vi "Utility_Translate circle into Masking ROI.vi"(11 "Fitted Circle":T2) -> (3 "ROI Descriptor":T1)   [LabVIEW 2014]
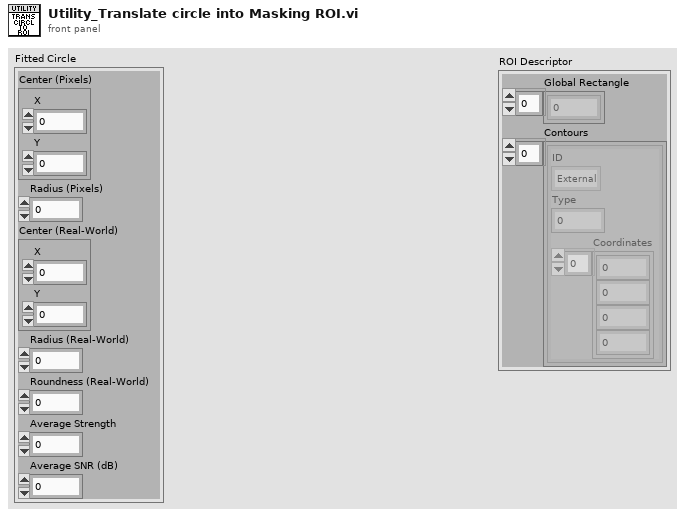
[diagram p1: front panel]
types:
  T1 = cluster{"Global Rectangle":i32[], "Contours":cluster{"ID":enum32{"External", "Internal"}, "Type":u32, "Coordinates":i32[]}[]}
  T2 = cluster{"Center (Pixels)":cluster{"X":sgl, "Y":sgl}, "Radius (Pixels)":dbl, "Center (Real-World)":cluster{"X":sgl, "Y":sgl}, "Radius (Real-World)":dbl, "Roundness (Real-World)":dbl, "Average Strength":dbl, "Average SNR (dB)":dbl}
  T3 = cluster{"ID":enum32{"External", "Internal"}, "Type":u32, "Coordinates":i32[]}
  T4 = cluster{"ID":enum32{"External", "Internal"}, "Type":u32, "Coordinates":i32[]}[]
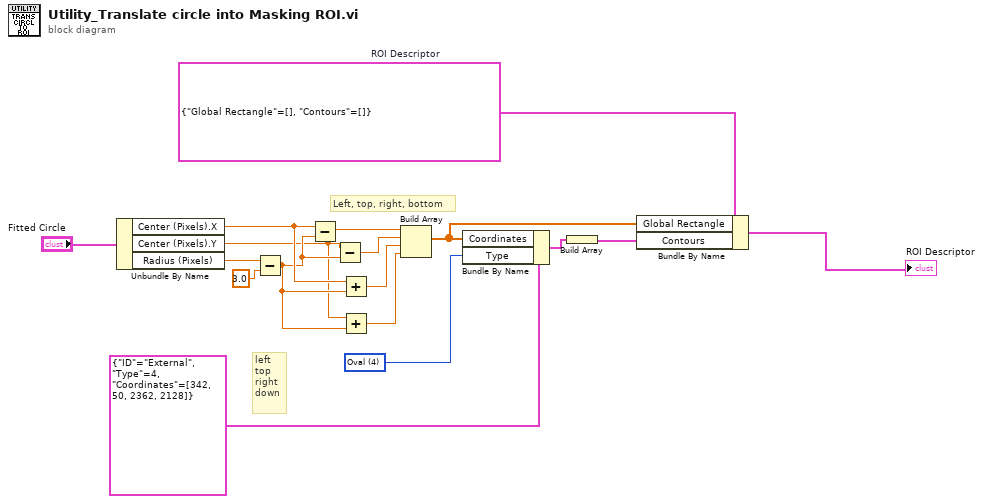
[diagram p0: block diagram]
diagram:
  w1 = u32 4 items=["No Selection", "Point", "Line", "Rectangle", "Oval", "Polygon", "Freehand Region", "Annulus", "Unused2", "Unused3", "Broken Line", "Freehand Line", "Rotated Rectangle"] ("Type")
  w14 = T1 {"Global Rectangle"=[], "Contours"=[]}  # ROI Descriptor
  # "Left, top, right, bottom"
  # "left \ntop\nright \ndown"
  n1 = Unbundle By Name("Fitted Circle") -> ("Center (Pixels).X"=w9:sgl, "Center (Pixels).Y"=w4:sgl, "Radius (Pixels)"=w11:dbl)
  n2 = Subtract(x=w11, y=3.0) -> (x-y=w8:dbl)
  n3 = Subtract(x=w9, y=w8) -> (x-y=w7:dbl)
  n4 = Subtract(x=w4, y=w8) -> (x-y=w6:dbl)
  n5 = Add(x=w9, y=w8) -> (x+y=w5:dbl)
  n6 = Add(x=w4, y=w8) -> (x+y=w2:dbl)
  n7 = Build Array(w7, w6, w5, w2) -> (w3:dbl[])
  n8 = Bundle By Name(cluster=T3 {"ID"=enum."External", "Type"=4, "Coordinates"=[342, 50, 2362, 2128]}, "Coordinates"=w3, "Type"=w1) -> (w15:T3)
  n9 = Build Array(w15) -> (w13:T4)
  n10 = Bundle By Name(cluster=w14, "Global Rectangle"=w3, "Contours"=w13) -> (→"ROI Descriptor":T1)
